vi "Set Decoration Tag.vi"(8 "error in (no error)":errorcluster, 11 "VI Refnum":refnum<vi>) -> (0 "error out":errorcluster)   [LabVIEW 2017]
uses:
  <vilib>/UserTags/UserTags.lvlib
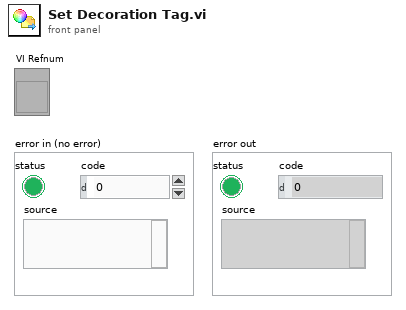
[diagram p1: front panel]
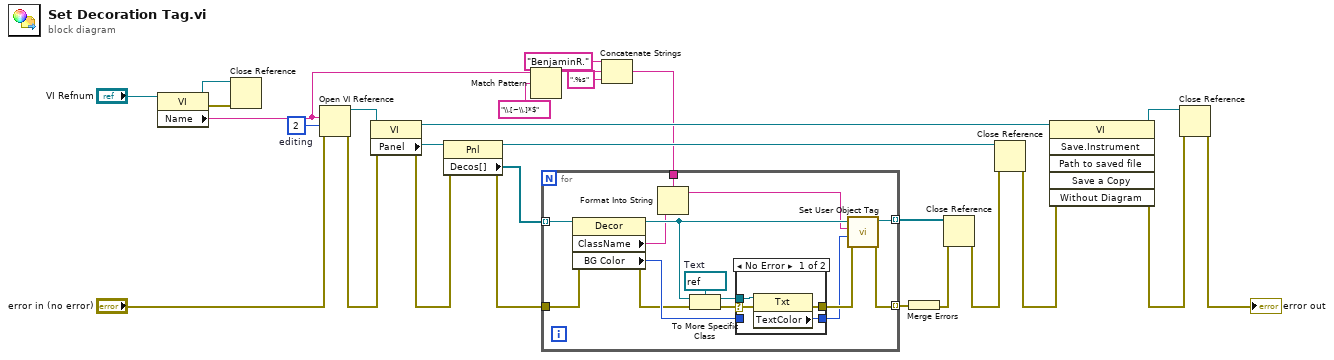
[diagram p0: block diagram]
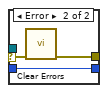
[diagram p2: hidden frame]
diagram:
  w27 = 2  # editing
  n1 = property class="VI"(reference="VI Refnum") -> (reference out=w23:refnum<vi>, error out=w24:errorcluster, "Name"=w6:string)  [unwired: 1 in]
  n2 = Close Reference(reference=w23, error in (no error)=w24) -> ()  [unwired: 1 out]
  n3 = Open VI Reference(vi path=w6, options=w27, error in (no error)="error in (no error)") -> (vi reference=w26:refnum<vi>, error out=w20:errorcluster)  [unwired: 3 in]
  n4 = property class="VI"(reference=w26, error in=w20) -> (reference out=w21:refnum<vi>, error out=w19:errorcluster, "Panel"=w25:refnum<vi>)
  n5 = property class="Pnl"(reference=w25, error in=w19) -> (reference out=w14:refnum<vi>, error out=w17:errorcluster, "Decos[]"=w22:refnum<vi>[])
  n6 = Match Pattern(string=w6, regular expression="\\.[~\\.]*$") -> (before substring=w4:string)  [unwired: 4 out]
  n7 = Concatenate Strings("BenjaminR." ("string"), w4, ".%s" ("string")) -> (w2:string)
  n8 = for {
    tunnel: w22 -> [w42] mode=indexing
    tunnel: w2 -> [w41]
    tunnel: [w34] -> w18 mode=indexing
    tunnel: w17 -> [w32]
    tunnel: [w31] -> w15 mode=indexing
    w39 = refnum<vi> refnum  # Text
    n9 = property class="Decor"(reference=w42, error in=w32) -> (reference out=w40:refnum<vi>, error out=w33:errorcluster, "ClassName"=w30:string, "BG Color"=w36:u32)
    n10 = Format Into String(format string=w41, w30) -> (resulting string=w28:string)  [unwired: 2 in, 1 out]
    n11 = To More Specific Class(target class=w39, reference=w40, error in=w33) -> (specific class reference=w38:refnum<vi>, error out=w37:errorcluster)
    n12 = case shown="No Error" w37 {
      selector: w37 -> [w43 w48]
      tunnel: w38 -> [w46 _]
      tunnel: w36 -> [_ w49]
      tunnel: [w45 w49] -> w29
      tunnel: [w44 w47] -> w35
      frame No Error {
        n13 = property class="Txt"(reference=w46, error in=w43) -> (error out=w44:errorcluster, "TextColor"=w45:u32)  [unwired: 1 out]
      }
      frame Error {
        n14 = call <vilib>:"Clear Errors.vi"("error in (no error)"=w48) -> ("error out"=w47:errorcluster)  [unwired: 5 in, 1 out]
      }
    }
    n15 = call <vilib>:"Set User Object Tag.vi"("error in (no error)"=w35, "Value"=w29, "Tag Name"=w28, "Generic Refnum"=w40) -> ("error out"=w34:errorcluster, "dup Generic Refnum"=w31:refnum<vi>)  [unwired: 5 in, 1 out]
  }
  n16 = Merge Errors(w18) -> (w12:errorcluster)
  n17 = Close Reference(reference=w15, error in (no error)=w12) -> (error out=w13:errorcluster)
  n18 = Close Reference(reference=w14, error in (no error)=w13) -> (error out=w11:errorcluster)
  n19 = invoke class="VI" method="Save.Instrument"(reference=w21, error in=w11) -> (reference out=w10:refnum<vi>, error out=w9:errorcluster)  [unwired: 4 in, 4 out]
  n20 = Close Reference(reference=w10, error in (no error)=w9) -> (error out=→"error out":errorcluster)
